vi "Register for Events.vi"(8 "error in (no error)":errorcluster, 11 "Execution API In":refnum<class "Execution API.lvclass">) -> (0 "error out":errorcluster, 2 "Event Registration":refnum<event-registration>, 3 "Execution API Out":refnum<class "Execution API.lvclass">)   [LabVIEW 2020, in "Execution API.lvclass"]
doc: "Obtain an event registration which can be used to observe the execution while running and obtain results."
uses:
  Execution API.lvclass
  Core/Result/Result.ctl
  Core/Result/Status.ctl
  Core/Result/Type.ctl
  Execution API.lvclass/Execution API.ctl
  Core/Result/Result.lvlib
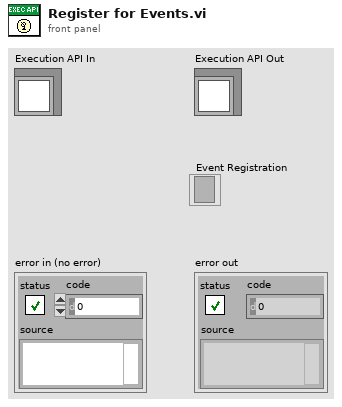
[diagram p1: front panel]
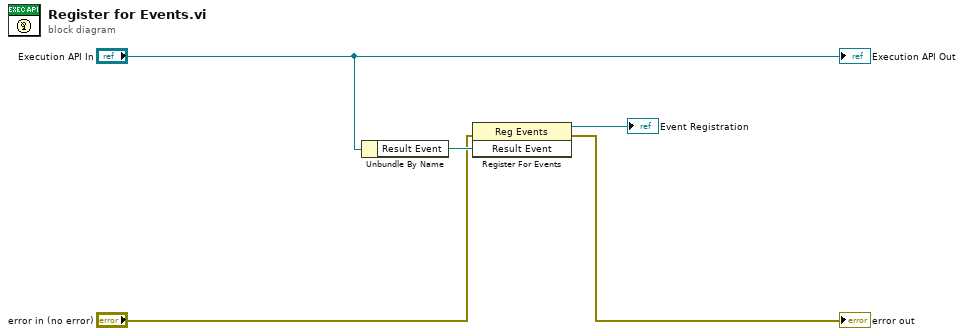
[diagram p0: block diagram]
diagram:
  n1 = Unbundle By Name("Execution API In") -> ("Result Event"=w4:refnum<user-event>)
  n2 = register-events(error in="error in (no error)", w4) -> (reference out=→"Event Registration":refnum<event-registration>, error out=→"error out":errorcluster)  [unwired: 1 in]
  "Execution API Out" <- "Execution API In"
